vi "prep bdd cloture.vi"(8 "tabin":string[](array[string]), 10 "seconds since 1Jan1904":timestamp, 11 "Ok final":bool) -> (0 "tabout":string[](array[string]))   [LabVIEW 2020]
uses:
  ctrl glo/selectdata.ctl
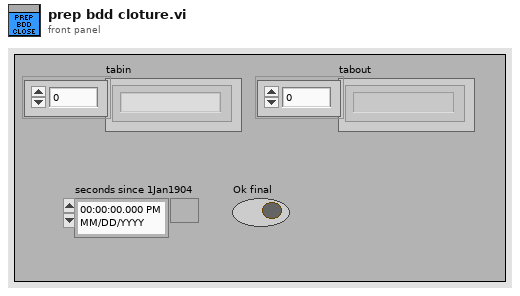
[diagram p1: front panel]
types:
  T1 = typedef "selectdata.ctl" = u16
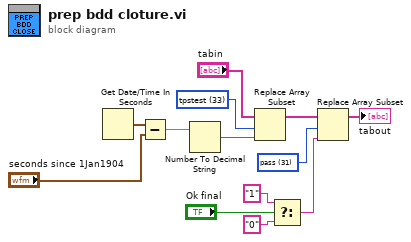
[diagram p0: block diagram]
diagram:
  w8 = T1 33 items=["id", "date", "type", "sn", "ocv", "acir", "insuP", "insuN", "TC01", "TC02", "TC11", "TC12", "TC21", "TC22", "VC01", "VC02", "VC03", "VC04", "VC11", "VC12", "VC13", "VC14", "VC21", "VC22", "VC23", "VC24", "DCIRN", "DCIRP", "inifilevers", "softvers", "imagevers", "pass", "operateur", "tpstest"] ("Menu déroulant")
  w1 = T1 31 items=["id", "date", "type", "sn", "ocv", "acir", "insuP", "insuN", "TC01", "TC02", "TC11", "TC12", "TC21", "TC22", "VC01", "VC02", "VC03", "VC04", "VC11", "VC12", "VC13", "VC14", "VC21", "VC22", "VC23", "VC24", "DCIRN", "DCIRP", "inifilevers", "softvers", "imagevers", "pass", "operateur", "tpstest"] ("Menu déroulant")
  n1 = Get Date/Time In Seconds() -> (seconds since 1Jan1904=w6:timestamp)
  n2 = Subtract(x=w6, y="seconds since 1Jan1904") -> (x-y=w11:dbl)
  n3 = Number To Decimal String(number=w11) -> (decimal integer string=w12:string)  [unwired: 1 in]
  n4 = Replace Array Subset(array="tabin", new element=w12, index=w8) -> (w10:string[])
  n5 = Select ("Sélectionner")(t="1", s="Ok final", f="0") -> (s? t:f=w5:string)
  n6 = Replace Array Subset(array=w10, new element=w5, index=w1) -> (→"tabout":string[])
